vi "Launcher.vi"   [LabVIEW 2011]
doc: "Is used to start main.vi from the same folder.\nShould be application startup vi.\n\nAlso used for setting the version"
uses:
  emi Lib/Basic/0 - General/App/Version/Private/emi_Version Info.ctl
  emi Lib/System 01/1 - GUI/Profiling Mar-In/Splash & About/Private/emi_Splash&About Screen.vi
panel:
  # "Is used to start main.vi from the same folder.\nShould be application startup vi."
types:
  T1 = enum32{"Invalid", "Standard", "Closed", "Hidden", "Minimized", "Maximized"}
  T2 = typedef "emi_Version Info.ctl" = cluster{"Name":string, "Major":i16, "Minor":i16, "Fix":i16, "Build":i32, "Type":enum16{"Alfa", "Beta", "Stable"}, "Dev":bool, "Version Name":string, "Date":timestamp}
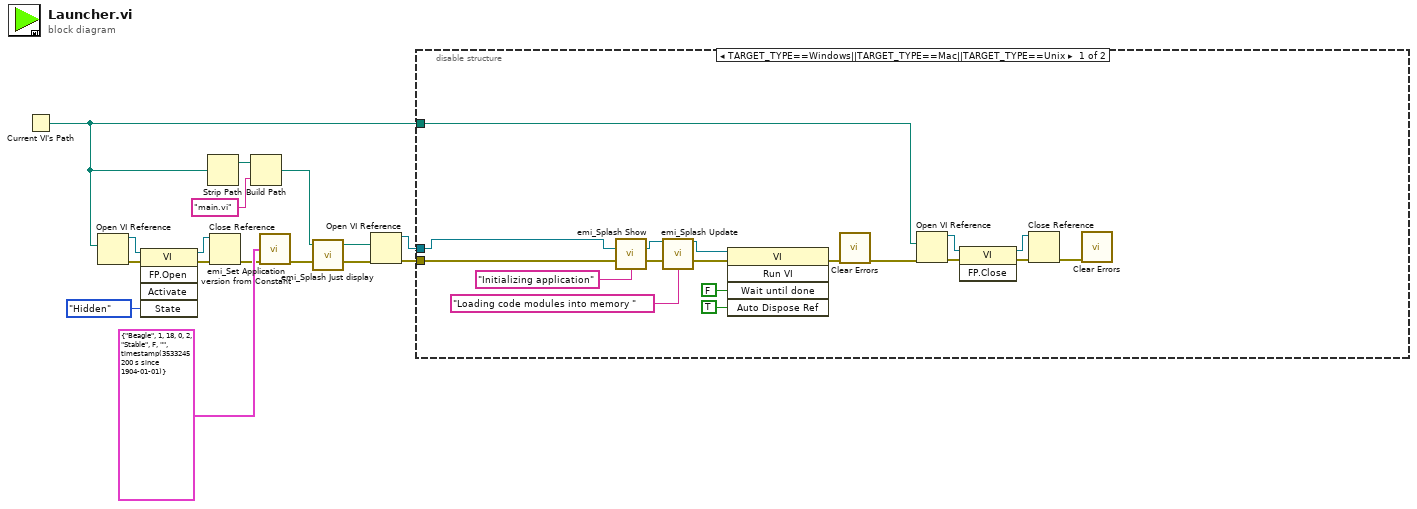
[diagram p0: block diagram]
diagram:
  n1 = Current VI's Path() -> (path=w5:path)
  n2 = Open VI Reference(vi path=w5) -> (vi reference=w8:refnum<vi>, error out=w11:errorcluster)  [unwired: 5 in]
  n3 = invoke class="VI" method="FP.Open"(reference=w8, error in=w11, "State"=T1."Hidden") -> (reference out=w7:refnum<vi>, error out=w9:errorcluster)  [unwired: 2 in, 3 out]
  n4 = Strip Path(path=w5) -> (stripped path=w13:path)  [unwired: 1 out]
  n5 = Close Reference(reference=w7, error in (no error)=w9) -> (error out=w2:errorcluster)
  n6 = Build Path(base path=w13, name or relative path="main.vi") -> (appended path=w14:path)
  n7 = call "emi_Set Application version from Constant.vi"("Version Info in"=T2 {"Name"="Beagle", "Major"=1, "Minor"=18, "Fix"=0, "Build"=2, "Type"=enum."Stable", "Dev"=FALSE, "Version Name"="", "Date"=timestamp(3533245200 s since 1904-01-01)}, "error in (no error)"=w2) -> ("error out"=w1:errorcluster)  [unwired: 12 in, 1 out]
  n8 = call "emi_Splash Just display.vi"("error In"=w1) -> ("error out"=w10:errorcluster)  [unwired: 13 in, 1 out]
  n9 = Open VI Reference(vi path=w14, error in (no error)=w10) -> (vi reference=w4:refnum<vi>, error out=w3:errorcluster)  [unwired: 4 in]
  n10 = disable-structure shown="TARGET_TYPE==Windows||TARGET_TYPE==Mac||TARGET_TYPE==Unix" {
    disable-tunnel: w3 -> [w18 _]
    disable-tunnel: w4 -> [w17 _]
    disable-tunnel: w5 -> [w21 _]
    frame condition #0 (active) {
      n11 = call "emi_Splash Show.vi"("Counter Refnum(Calling VI)"=w17, "error In"=w18, "Status text"="Initializing application") -> ("Counter Refnum out"=w16:refnum<vi>, "error out"=w32:errorcluster)  [unwired: 11 in]
      n12 = call "emi_Splash Update.vi"("error In"=w32, "Task Text"="Loading code modules into memory ") -> ("error out"=w29:errorcluster)  [unwired: 13 in]
      n13 = invoke class="VI" method="Run VI"(reference=w16, error in=w29, "Wait until done"=FALSE ("Wait Until Done"), "Auto Dispose Ref"=TRUE ("Auto Dispose Reference")) -> (error out=w26:errorcluster)  [unwired: 1 in, 4 out]
      n14 = call <vilib>:"Clear Errors.vi"("error in (no error)"=w26) -> ("error out"=w20:errorcluster)  [unwired: 6 in]
      n15 = Open VI Reference(vi path=w21, error in (no error)=w20) -> (vi reference=w24:refnum<vi>, error out=w22:errorcluster)  [unwired: 4 in]
      n16 = invoke class="VI" method="FP.Close"(reference=w24, error in=w22) -> (reference out=w25:refnum<vi>, error out=w23:errorcluster)  [unwired: 1 in, 1 out]
      n17 = Close Reference(reference=w25, error in (no error)=w23) -> (error out=w19:errorcluster)
      n18 = call <vilib>:"Clear Errors.vi"("error in (no error)"=w19) -> ()  [unwired: 6 in, 1 out]
    }
    frame condition #1 {
    }
  }
